vi "Actor Core.vi"(8 "error in (no error)":errorcluster, 11 "Mag Lab Measure Interface in":refnum<class "MagLabGraph.lvclass">) -> (0 "error out":errorcluster, 3 "Actor Framework.lvlib:Actor":refnum<class "Actor.lvclass">)   [LabVIEW 2015, in "MagLabGraph.lvclass"]
uses:
  MagLabGraph.lvclass
  <vilib>/ActorFramework/Actor/Actor.lvclass
  MagLabGraph.lvclass/MagLabGraph.ctl
  <vilib>/ActorFramework/Actor/Actor.lvclass/Actor.ctl
  <vilib>/ActorFramework/Message Enqueuer/Message Enqueuer.lvclass/Message Enqueuer.ctl
  Mag Lab Measure Base Messages/Graph Closed Msg/Graph Closed Msg.lvclass/Graph Closed Msg.ctl
  MagLabGraph Messages/Add file Msg/Add file Msg.lvclass/Add file Msg.ctl
  <vilib>/ActorFramework/Message Enqueuer/Init from Existing Queue.vi
  <vilib>/ActorFramework/Message Enqueuer/Enqueue.vi
  <vilib>/ActorFramework/Message Priority Queue/Priority Enqueue.vi
  Mag Lab Error Handler/Send Error.vi
  <vilib>/ActorFramework/Message Enqueuer/Message Enqueuer.lvclass
  <vilib>/ActorFramework/Stop Msg/Stop Msg.lvclass
  Mag Lab Measure Base Messages/Graph Closed Msg/Graph Closed Msg.lvclass
  MagLabGraph Messages/Add file Msg/Add file Msg.lvclass
  MagLabGraph Messages/Save keep old plots Msg/Save keep old plots Msg.lvclass
  MagLabGraph Messages/Replot Msg/Replot Msg.lvclass
  MagLabGraph Messages/Save defaults Msg/Save defaults Msg.lvclass
  Mag Lab Measure Interface/Mag Lab Measure UI.lvclass
panel:
  in  "Set as default":bool
  in  "Keep old\nplots":bool
  in  "Open":bool
  in  "Exit":bool
  in  "Plots":cluster{"X":u16, "Y":u16}[](array[cluster]) {"Y" items=["Select channel...", "Time", "Y"]; "X" items=["Select channel...", "Time", "Y"]}
  out "XY Graph":cluster{dbl[], dbl[]}[](graph)
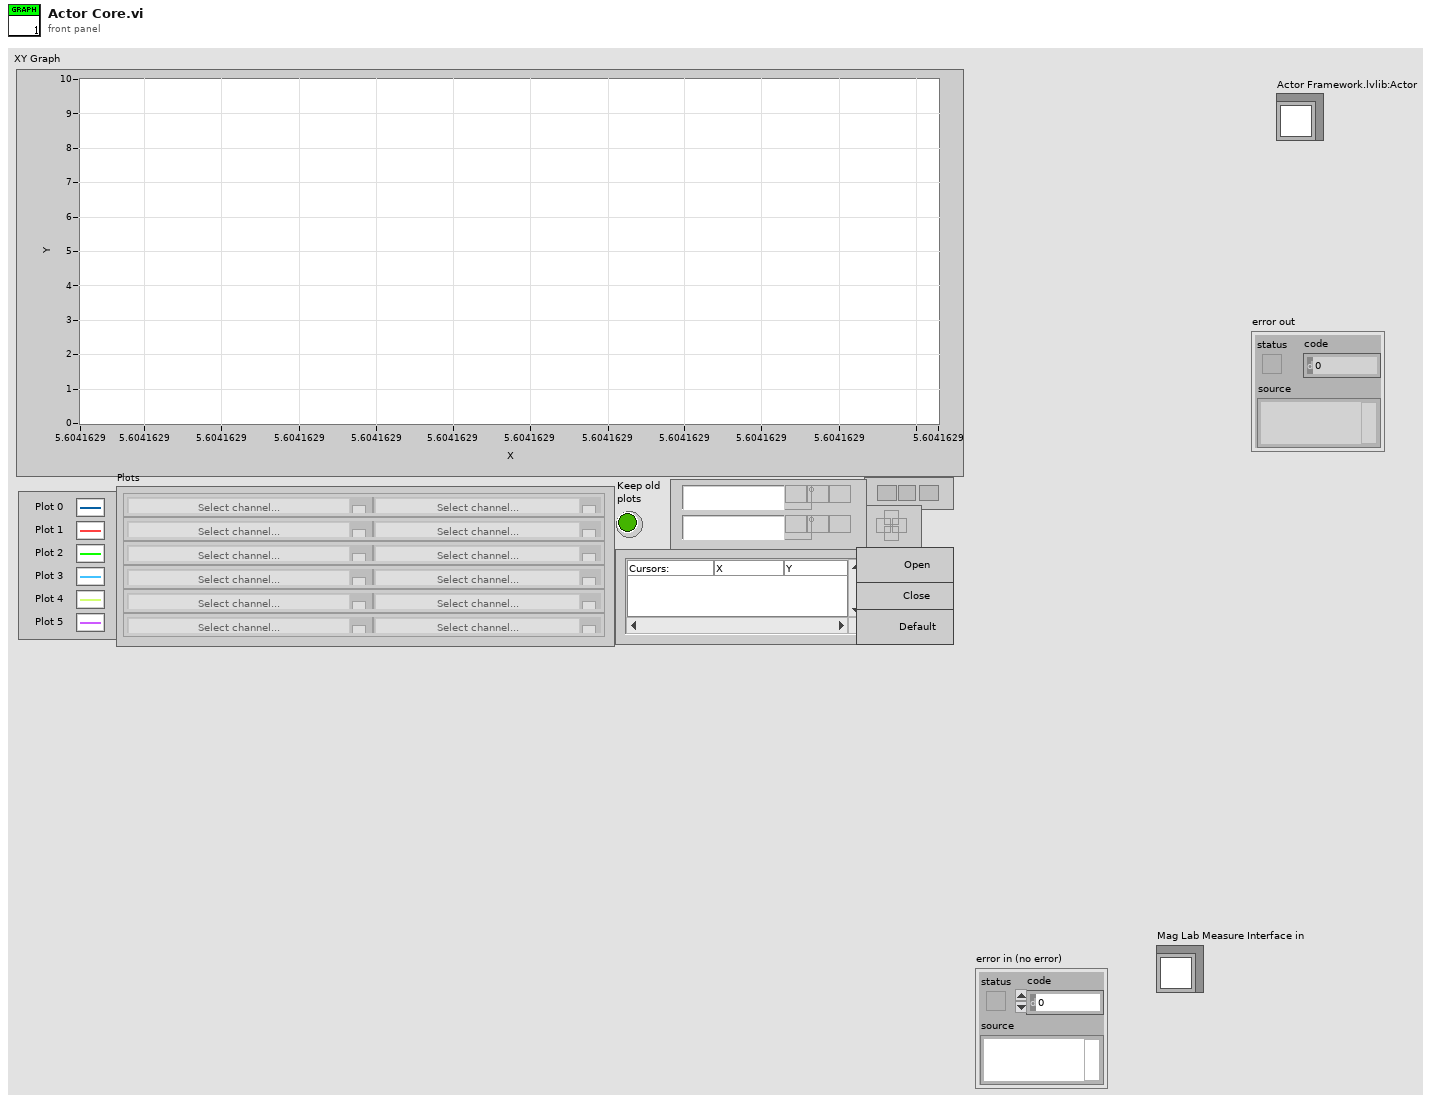
[diagram p1: front panel]
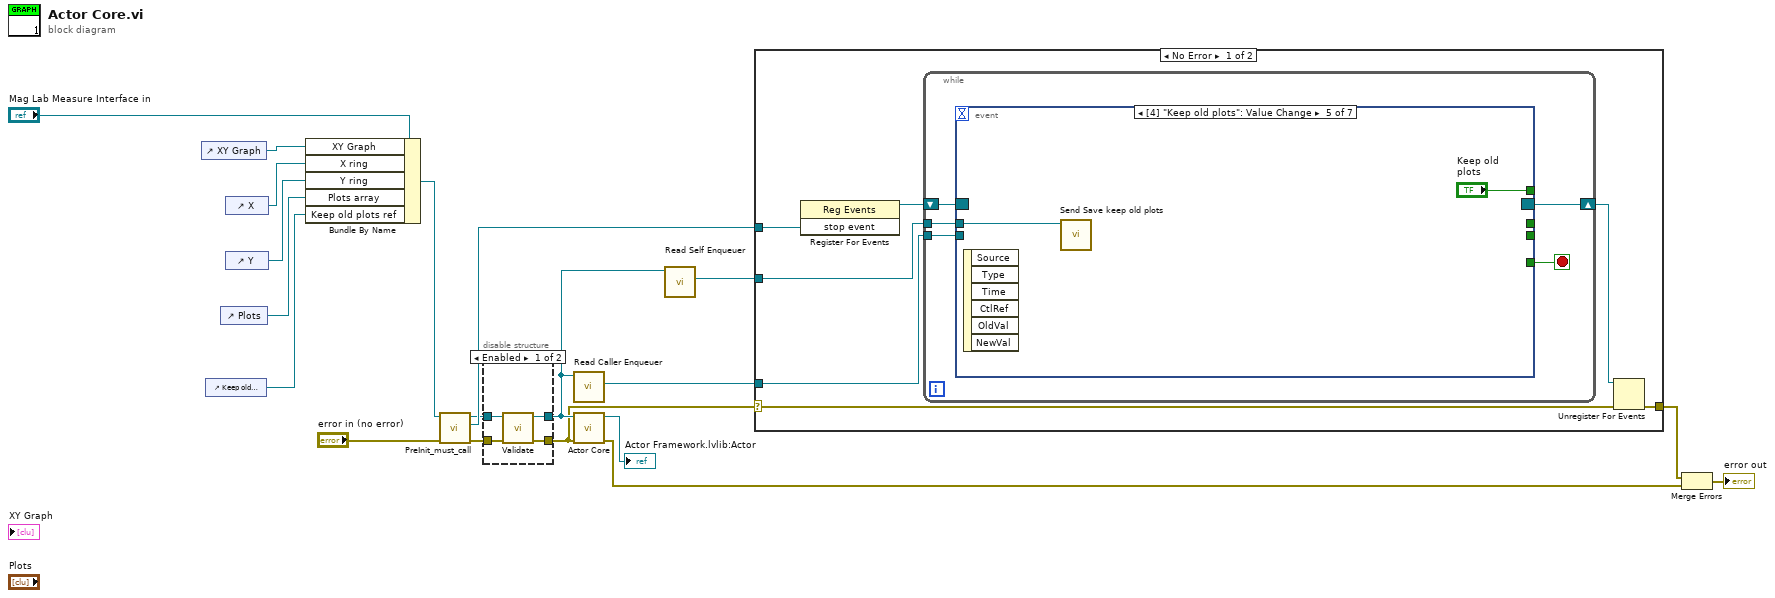
[diagram p0: block diagram]
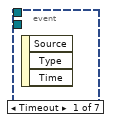
[diagram p3: hidden frame]
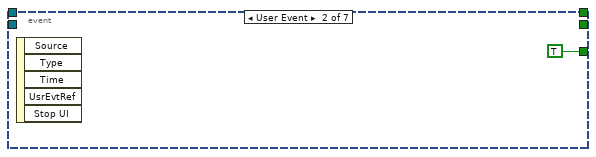
[diagram p4: hidden frame]
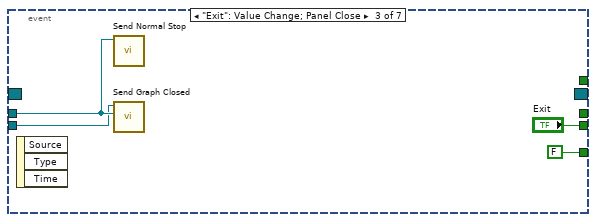
[diagram p5: hidden frame]
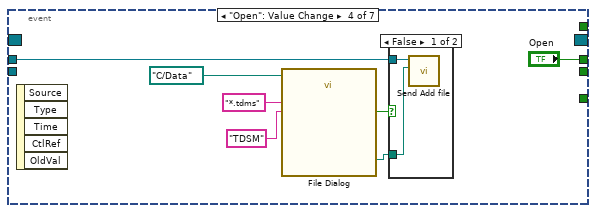
[diagram p6: hidden frame]
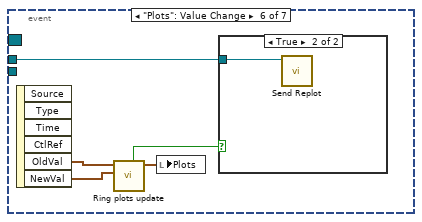
[diagram p8: hidden frame]
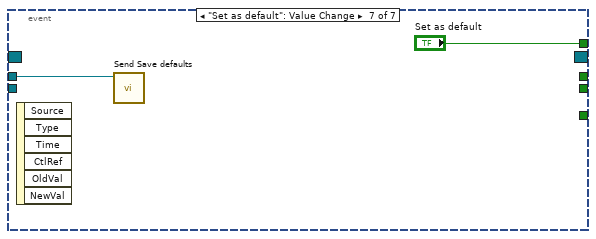
[diagram p10: hidden frame]
diagram:
  n1 = control-ref of="XY Graph"() -> (w9:refnum<vi>)
  n2 = control-ref of="Keep old\nplots"() -> (w4:refnum<vi>)
  n3 = control-ref of="Plots"() -> (w13:refnum<vi>)
  n4 = control-ref of="X"() -> (w12:refnum<vi>)
  n5 = control-ref of="Y"() -> (w11:refnum<vi>)
  n6 = Bundle By Name(cluster="Mag Lab Measure Interface in", "XY Graph"=w9, "X ring"=w12, "Y ring"=w11, "Plots array"=w13, "Keep old plots ref"=w4) -> (w14:refnum<class "MagLabGraph.lvclass">)
  n7 = call-dynamic "PreInit_must_call.vi"("error in (no error)"="error in (no error)", "Mag Lab Measure Interface in"=w14) -> ("error out"=w6:errorcluster, "stop event"=w18:refnum<user-event>, "Mag Lab Measure Interface out"=w5:refnum<class "MagLabGraph.lvclass">)  [unwired: 7 in]
  n8 = disable-structure shown="Enabled" {
    disable-tunnel: [w23 w25] -> w3
    disable-tunnel: [w22 w24] -> w7
    disable-tunnel: w6 -> [w21 w25]
    disable-tunnel: w5 -> [w20 w24]
    frame Enabled {
      n9 = call-dynamic "Validate.vi"("error in (no error)"=w21, "MagLabGraph in"=w20) -> ("error out"=w23:errorcluster, "MagLabGraph out"=w22:refnum<class "MagLabGraph.lvclass">)  [unwired: 8 in]
    }
    frame Disabled {
    }
  }
  n10 = call <vilib>:"Read Caller Enqueuer.vi"("Actor"=w7) -> ("Caller Enqueuer"=w8:refnum<class "Message Enqueuer.lvclass">)  [unwired: 10 in]
  n11 = call-parent "Actor Core.vi"("error in (no error)"=w3, "Mag Lab Measure Interface in"=w7) -> ("error out"=w1:errorcluster, "Actor Framework.lvlib:Actor"=→"Actor Framework.lvlib:Actor":refnum<class "Actor.lvclass">)  [unwired: 8 in]
  n12 = call <vilib>:"Read Self Enqueuer.vi"("Actor"=w7) -> ("Self Enqueuer"=w16:refnum<class "Message Enqueuer.lvclass">)  [unwired: 10 in]
  n13 = case shown="No Error" w3 {
    selector: w3 -> [w26 w62]
    tunnel: w18 -> [w31 _]
    tunnel: w16 -> [w30 _]
    tunnel: [w29 w62] -> w15
    tunnel: w8 -> [w27 _]
    frame No Error {
      n14 = register-events(w31) -> (reference out=w32:refnum<event-registration>)  [unwired: 2 in, 1 out]
      n15 = while {
        tunnel: w30 -> [w36]
        shift-right: [w34] -> w28
        shift-left: w32 -> [w37]
        tunnel: w27 -> [w33]
        stop <- w35 stop-if-true
        n16 = event shown="[4] \"Keep old plots\": Value Change" {
          selector: w37 -> [_ _ _ _ _ _ _]
          dyn-events: [_ _ _ _ _ _ _] -> w34
          timeout: _ -> [_ _ _ _ _ _ _]
          tunnel: w36 -> [_ _ w40 w44 w53 w54 w60]
          tunnel: [_ TRUE FALSE _ _ _ _] -> w35
          tunnel: [_ _ "Exit" _ _ _ _] -> _
          tunnel: [_ _ _ "Open" _ _ _] -> _
          tunnel: w33 -> [_ _ w39 _ _ _ _]
          tunnel: [_ _ _ _ "Keep old\nplots" _ "Set as default"] -> _
          event Timeout {
            n17 = event-data() -> ()  [unwired: 1 in, 3 out]
          }
          event User Event {
            n18 = event-data() -> ()  [unwired: 1 in, 5 out]
          }
          event "Exit": Value Change; Panel Close {
            n19 = event-data() -> ()  [unwired: 1 in, 3 out]
            n20 = call <vilib>:"Send Normal Stop.vi"("Message Enqueuer"=w40) -> ()  [unwired: 10 in, 1 out]
            n21 = call "Send Graph Closed.vi"("Closed Graph"=w40, "Message Enqueuer"=w39) -> ()  [unwired: 8 in, 2 out]
          }
          event "Open": Value Change {
            n22 = event-data() -> ()  [unwired: 1 in, 5 out]
            n23 = call "File Dialog"("start path"=path "C:/Data", "pattern (all files)"="*.tdms", "pattern label"="TDSM") -> ("selected path"=w43:path, "cancelled"=w45:bool)  [unwired: 9 in, 2 out]
            n24 = case shown="False" w45 {
              tunnel: w44 -> [w51 _]
              tunnel: w43 -> [w50 _]
              frame False {
                n25 = call "Send Add file.vi"("File Path Control"=w50, "Message Enqueuer"=w51) -> ()  [unwired: 8 in, 2 out]
              }
              frame True {
              }
            }
          }
          event "Keep old\nplots": Value Change {
            n26 = event-data() -> ()  [unwired: 1 in, 6 out]
            n27 = call "Send Save keep old plots.vi"("Message Enqueuer"=w53) -> ()  [unwired: 9 in, 2 out]
          }
          event "Plots": Value Change {
            n28 = event-data() -> ("OldVal"=w56:cluster{"X":u16, "Y":u16}[], "NewVal"=w57:cluster{"X":u16, "Y":u16}[])  [unwired: 1 in, 4 out]
            n29 = call "Ring plots update.vi"("New Plots"=w57, "Old Plots"=w56) -> ("Plots"=w58:cluster{"X":u16, "Y":u16}[], "Replot?"=w55:bool)  [unwired: 8 in]
            n30 = local write "Plots"(w58) -> ()
            n31 = case shown="True" w55 {
              tunnel: w54 -> [_ w59]
              frame False {
              }
              frame True {
                n32 = call "Send Replot.vi"("Message Enqueuer"=w59) -> ()  [unwired: 9 in, 2 out]
              }
            }
          }
          event "Set as default": Value Change {
            n33 = event-data() -> ()  [unwired: 1 in, 6 out]
            n34 = call "Send Save defaults.vi"("Message Enqueuer"=w60) -> ()  [unwired: 9 in, 2 out]
          }
        }
      }
      n35 = Unregister For Events(event registration refnum=w28, error in=w26) -> (error out=w29:errorcluster)
    }
    frame Error {
    }
  }
  n36 = Merge Errors(w15, w1) -> (→"error out":errorcluster)
